vi "Read Synthesizer Mode.vi"(11 "Signal Generator in":refnum<class "Signal Generator.lvclass">) -> (2 "Synthesizer Mode":enum16{"Normal", "Low Noise"}(ring), 3 "Signal Generator out":refnum<class "Signal Generator.lvclass">)   [LabVIEW 2020, in "Signal Generator.lvclass"]
uses:
  Signal Generator.lvclass
  Signal Generator.lvclass/Signal Generator.ctl
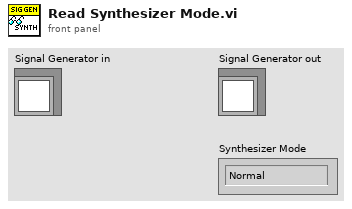
[diagram p1: front panel]
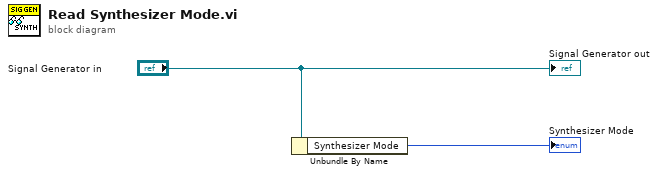
[diagram p0: block diagram]
diagram:
  n1 = Unbundle By Name("Signal Generator in") -> ("Synthesizer Mode"=→"Synthesizer Mode":enum16{"Normal", "Low Noise"})
  "Signal Generator out" <- "Signal Generator in"
